vi "5.vi"() -> ()   [LabVIEW 2017]
panel:
  in  "停止":bool
  out "油量报警":T1
  in  "控制面板":T2 {"档位" scale=0.0..6.0; "油门" scale=0.0..10.0}
  out "显示面板":T3 {"油量" scale=0.0..200.0; "速度（km/h）" scale=0.0..300.0; "转速（R/S）" scale=0.0..8000.0}
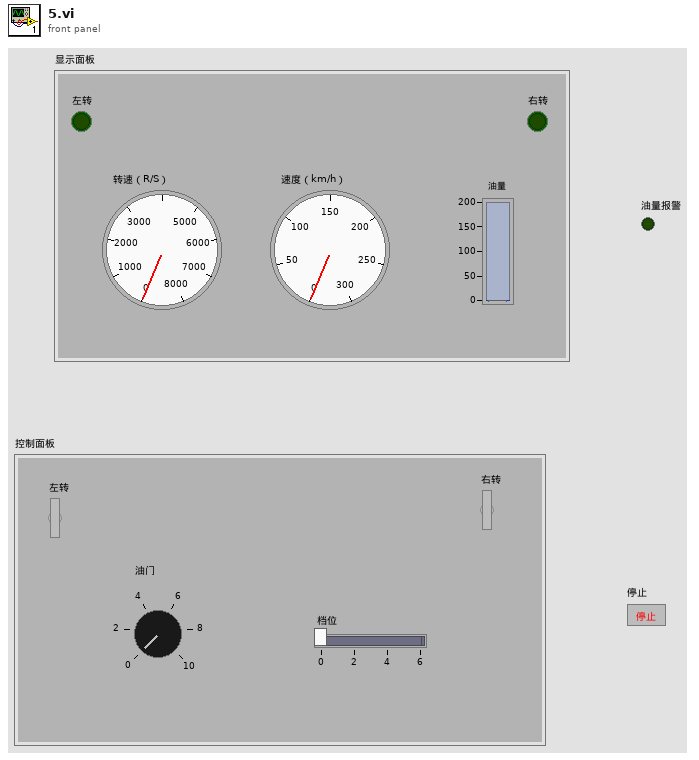
[diagram p1: front panel]
types:
  T1 = typedef "控件 1.ctl" = bool
  T2 = cluster{"左转":bool, "右转":bool, "油门":dbl, "档位":dbl}
  T3 = cluster{"左转":bool, "右转":bool, "转速（R/S）":dbl, "速度（km/h）":dbl, "油量":dbl}
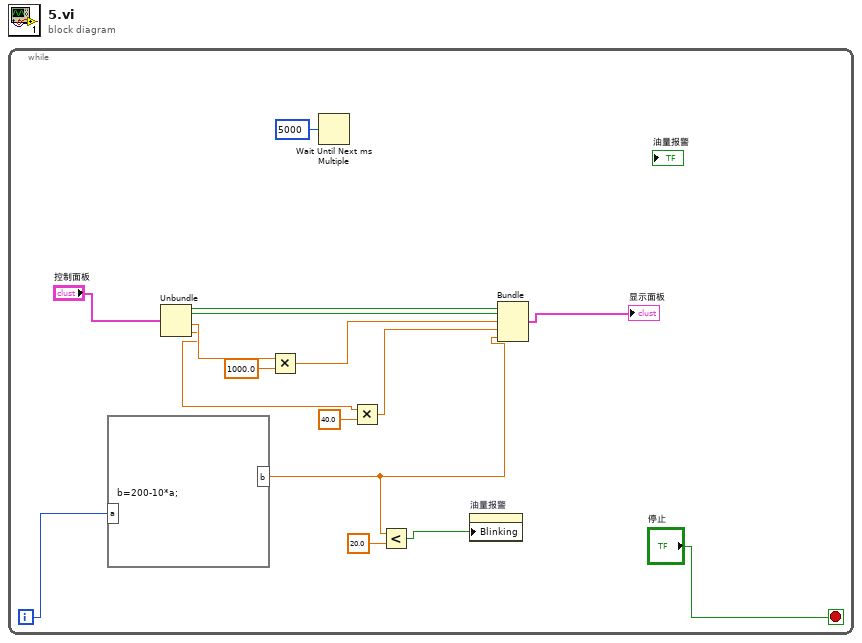
[diagram p0: block diagram]
diagram:
  n1 = while {
    i -> [w14]
    stop <- "停止" stop-if-true
    n2 = formula code="b=200-10*a;"("a"=w14) -> ("b"=w5:dbl)
    n3 = Unbundle("控制面板") -> ("左转"=w15:bool, "右转"=w2:bool, "油门"=w13:dbl, "档位"=w10:dbl)
    n4 = Multiply(x=w13, y=1000.0) -> (x*y=w11:dbl)
    n5 = Wait Until Next ms Multiple(millisecond multiple=u32 5000 ("毫秒倍数")) -> ()  [unwired: 1 out]
    n6 = Multiply(x=w10, y=40.0) -> (x*y=w8:dbl)
    n7 = Less?(x=w5, y=20.0) -> (x < y?=w4:bool)
    n8 = property on="油量报警" class="Bool (严格)"("Blinking"=w4) -> ()  [unwired: 2 in, 2 out]
    n9 = Bundle("左转"=w15, "右转"=w2, w11, w8, "b"=w5) -> (→"显示面板":cluster{"左转":bool, "右转":bool, dbl, dbl, "b":dbl})  [unwired: 1 in]
  }
